vi "subVI_saveParameters_demoinfocom.vi"   [LabVIEW 2021]
uses:
  USRP Channel Correlation/system stop.vi
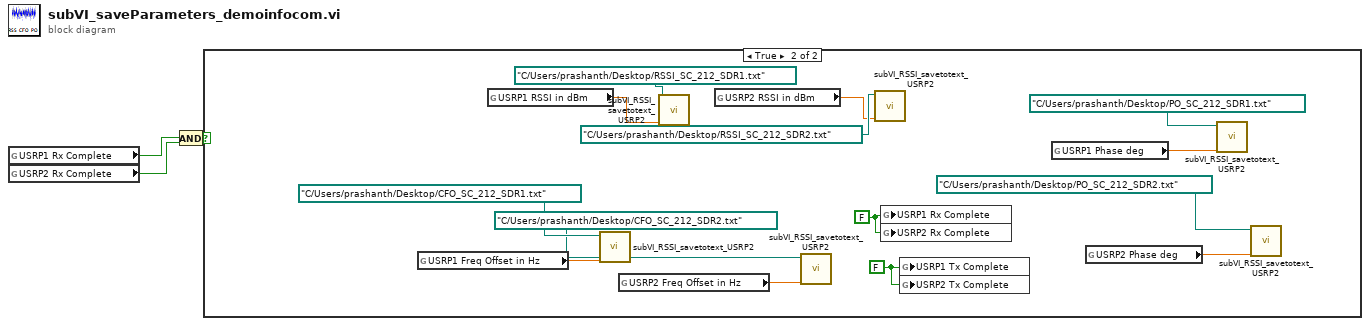
[diagram p0: block diagram]
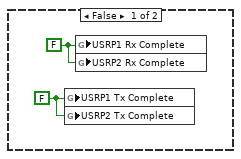
[diagram p2: hidden frame]
diagram:
  n1 = global read "system stop.vi" "USRP1 Rx Complete"() -> (w1:bool)
  n2 = global read "system stop.vi" "USRP2 Rx Complete"() -> (w2:bool)
  n3 = And(x=w1, y=w2) -> (x .and. y?=w3:bool)
  n4 = case shown="True" w3 {
    frame False {
      w5 = FALSE
      w4 = FALSE
      n5 = global write "system stop.vi" "USRP1 Tx Complete"(w5) -> ()
      n6 = global write "system stop.vi" "USRP2 Tx Complete"(w5) -> ()
      n7 = global write "system stop.vi" "USRP1 Rx Complete"(w4) -> ()
      n8 = global write "system stop.vi" "USRP2 Rx Complete"(w4) -> ()
    }
    frame True {
      w19 = FALSE
      w18 = FALSE
      n9 = global read "system stop.vi" "USRP1 Freq Offset in Hz"() -> (w12:dbl)
      n10 = global read "system stop.vi" "USRP1 RSSI in dBm"() -> (w16:dbl)
      n11 = call "subVI_RSSI_savetotext_USRP2.vi"("RSSI"=w12, "file path (dialog if empty)"=path "C:/Users/prashanth/Desktop/CFO_SC_212_SDR1.txt") -> ()  [unwired: 10 in]
      n12 = global read "system stop.vi" "USRP2 Freq Offset in Hz"() -> (w10:dbl)
      n13 = call "subVI_RSSI_savetotext_USRP2.vi"("RSSI"=w16, "file path (dialog if empty)"=path "C:/Users/prashanth/Desktop/RSSI_SC_212_SDR1.txt") -> ()  [unwired: 10 in]
      n14 = global read "system stop.vi" "USRP2 RSSI in dBm"() -> (w14:dbl)
      n15 = call "subVI_RSSI_savetotext_USRP2.vi"("RSSI"=w10, "file path (dialog if empty)"=path "C:/Users/prashanth/Desktop/CFO_SC_212_SDR2.txt") -> ()  [unwired: 10 in]
      n16 = call "subVI_RSSI_savetotext_USRP2.vi"("RSSI"=w14, "file path (dialog if empty)"=path "C:/Users/prashanth/Desktop/RSSI_SC_212_SDR2.txt") -> ()  [unwired: 10 in]
      n17 = global write "system stop.vi" "USRP1 Rx Complete"(w18) -> ()
      n18 = global write "system stop.vi" "USRP2 Rx Complete"(w18) -> ()
      n19 = global write "system stop.vi" "USRP1 Tx Complete"(w19) -> ()
      n20 = global write "system stop.vi" "USRP2 Tx Complete"(w19) -> ()
      n21 = global read "system stop.vi" "USRP1 Phase deg"() -> (w8:dbl)
      n22 = global read "system stop.vi" "USRP2 Phase deg"() -> (w6:dbl)
      n23 = call "subVI_RSSI_savetotext_USRP2.vi"("RSSI"=w8, "file path (dialog if empty)"=path "C:/Users/prashanth/Desktop/PO_SC_212_SDR1.txt") -> ()  [unwired: 10 in]
      n24 = call "subVI_RSSI_savetotext_USRP2.vi"("RSSI"=w6, "file path (dialog if empty)"=path "C:/Users/prashanth/Desktop/PO_SC_212_SDR2.txt") -> ()  [unwired: 10 in]
    }
  }
